vi "AES Encrypt.vi"(5 "Key":u8[](array[numeric]), 7 "IV":u8[](array[numeric]), 8 "error in (no error)":errorcluster, 10 "data":u8[](array[numeric]), 11 "AES in":refnum<class "AES.lvclass">) -> (0 "error out":errorcluster, 2 "encrypted_data":u8[](array[numeric]), 3 "AES out":refnum<class "AES.lvclass">)   [LabVIEW 2023, in "AES.lvclass"]
uses:
  AES.lvclass
  AES.lvclass/AES.ctl
  System.Core
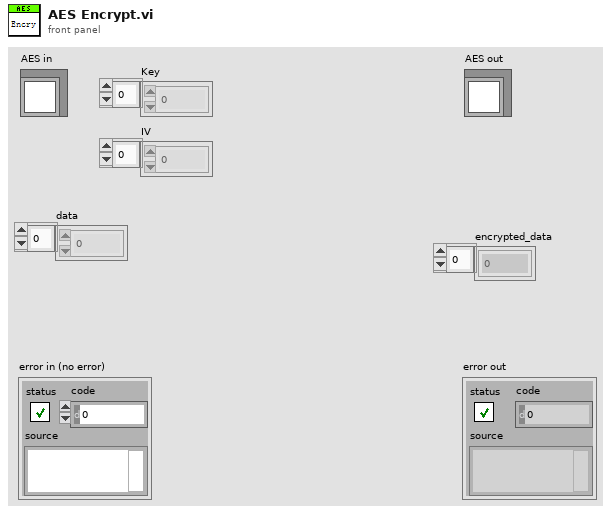
[diagram p1: front panel]
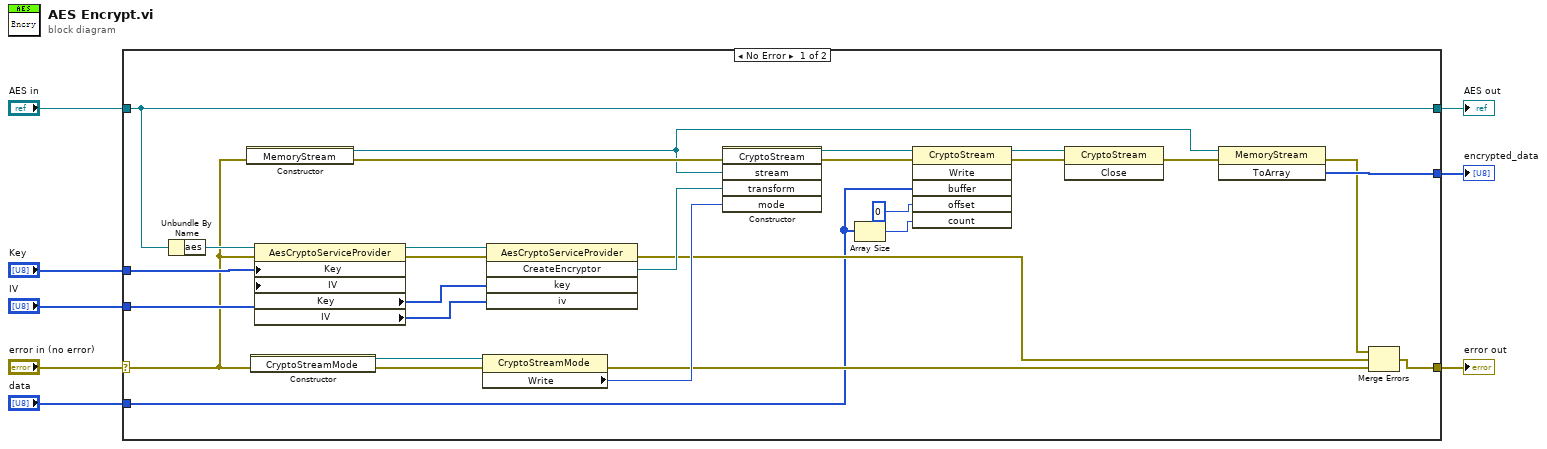
[diagram p0: block diagram]
diagram:
  n1 = case shown="No Error" "error in (no error)" {
    selector: "error in (no error)" -> [w27 w38]
    tunnel: [w10 w38] -> w7
    tunnel: [w32 w37] -> w5
    tunnel: "AES in" -> [w32 w37]
    tunnel: "Key" -> [w30 _]
    tunnel: "IV" -> [w29 _]
    tunnel: [w14 _] -> w2
    tunnel: "data" -> [w9 _]
    frame No Error {
      n2 = Unbundle By Name(w32) -> ("aes"=w31:refnum<k24>)
      n3 = constructor class="MemoryStream" ("AliceEntschlüsselt")(error in=w27) -> (reference out=w15:refnum<k24>, error out=w25:errorcluster)  [unwired: 2 in, 1 out]
      n4 = constructor class="CryptoStreamMode" ("AliceEntschlüsselt")(error in=w27) -> (reference out=w28:refnum<k24>, error out=w26:errorcluster)  [unwired: 2 in, 1 out]
      n5 = property class="AesCryptoServiceProvider"(reference=w31, error in=w27, "Key"=w30, "IV"=w29) -> (reference out=w35:refnum<k24>, error out=w36:errorcluster, "Key"=w34:u8[], "IV"=w33:u8[])
      n6 = property class="CryptoStreamMode"(reference=w28, error in=w26) -> (error out=w13:errorcluster, "Write"=w23:i32)  [unwired: 1 out]
      n7 = invoke class="AesCryptoServiceProvider" method="CreateEncryptor"(reference=w35, error in=w36, "key"=w34, "iv"=w33) -> (error out=w12:errorcluster, "CreateEncryptor"=w24:refnum<k24>)  [unwired: 1 in, 3 out]
      n8 = constructor class="CryptoStream" ("AliceEntschlüsselt")(error in=w25, "stream"=w15, "transform"=w24, "mode"=w23) -> (reference out=w21:refnum<k24>, error out=w22:errorcluster)  [unwired: 2 in, 4 out]
      n9 = Array Size(array=w9) -> (size(s)=w19:i32)
      n10 = invoke class="CryptoStream" method="Write"(reference=w21, error in=w22, "buffer"=w9, "offset"=0, "count"=w19) -> (reference out=w17:refnum<k24>, error out=w18:errorcluster)  [unwired: 1 in, 4 out]
      n11 = invoke class="CryptoStream" method="Close"(reference=w17, error in=w18) -> (error out=w16:errorcluster)  [unwired: 1 in, 2 out]
      n12 = invoke class="MemoryStream" method="ToArray"(reference=w15, error in=w16) -> (error out=w11:errorcluster, "ToArray"=w14:u8[])  [unwired: 1 in, 1 out]
      n13 = Merge Errors(w11, w12, w13) -> (w10:errorcluster)
    }
    frame Error {
    }
  }
  "error out" <- w7
  "AES out" <- w5
  "encrypted_data" <- w2
